vi "Labspec MoveMotor.vi"(6 "Position Name":string, 7 "Modes":T1[](array[typedef]) items=["Value"=0, "Step"=1, "Index"=2, "String"=3, "Calibrate"=4, "Origin"=5, "Stop"=6, "Value to Step"=7, "No Wait"=10, "No Message"=100], 8 "error in":errorcluster, 9 "Position Value":dbl=1.0, 10 "Motor Name":T2=enum."Hole", 11 "Automation Refnum In":refnum<k7>) -> (0 "error out":errorcluster, 2 "MoveID":i32, 3 "Automation Refnum Out":refnum<k7>)   [LabVIEW 2014]
uses:
  MoveMotor Motor Name.ctl
  MoveMotor Mode.ctl
panel:
  in  "Motor type (as in documentation)":u16(ring)=6 items=["Spectro", "Mono", "Grating", "Slit", "Hole", "X", "Y", "Z", "Laser"]
  # "LICENSED MATERIALS – PROPERTY OF IBM\nCopyright IBM Corp. 2016,\nALL RIGHTS RESERVED"
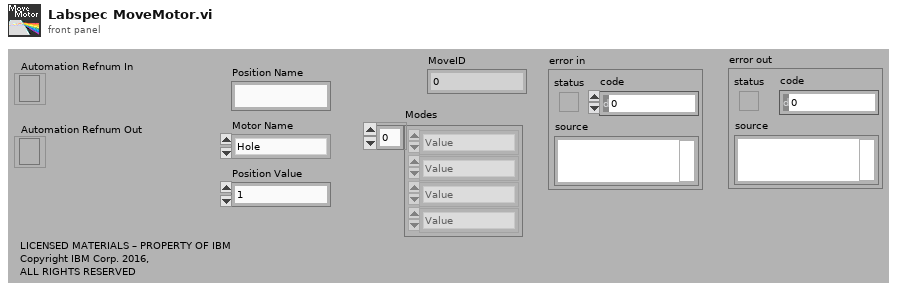
[diagram p1: front panel]
types:
  T1 = typedef "MoveMotor Mode.ctl" = u16
  T2 = typedef "MoveMotor Motor Name.ctl" = enum16{"Spectro", "Premono", "Grating", "Slit", "Hole", "X", "Y", "XT", "YT", "XL", "YL", "Z", "Laser", "Filter", "Objective", "Detector", "Detector Temperature"}
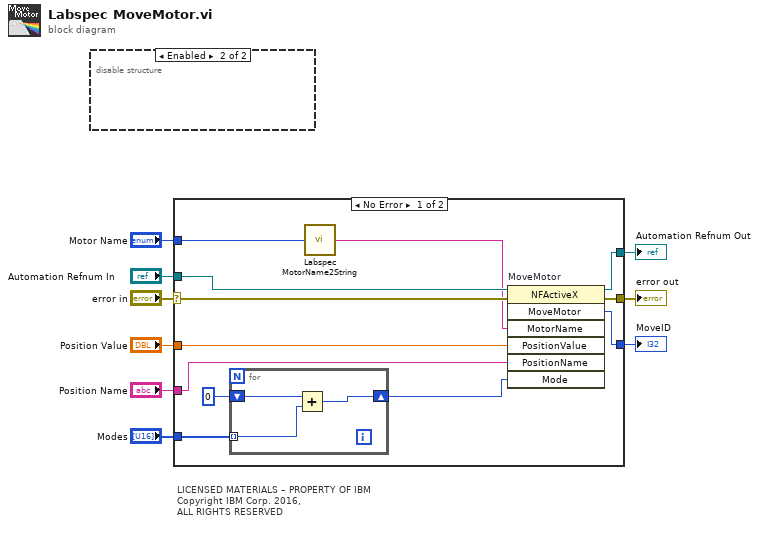
[diagram p0: block diagram]
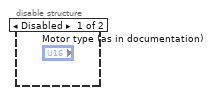
[diagram p2: hidden frame]
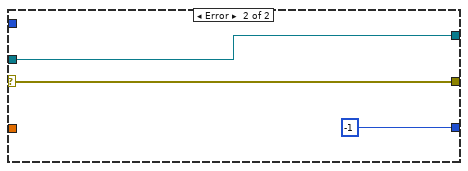
[diagram p3: hidden frame]
diagram:
  # "LICENSED MATERIALS – PROPERTY OF IBM\nCopyright IBM Corp. 2016,\nALL RIGHTS RESERVED"
  n1 = disable-structure shown="Enabled" {
    frame Disabled {
    }
    frame Enabled {
    }
  }
  n2 = case shown="No Error" "error in" {
    selector: "error in" -> [w15 w25]
    tunnel: "Modes" -> [w12 _]
    tunnel: "Position Name" -> [w21 _]
    tunnel: [w20 -1 ("MoveMotor")] -> w8
    tunnel: "Position Value" -> [w19 _]
    tunnel: "Motor Name" -> [w14 _]
    tunnel: "Automation Refnum In" -> [w18 w27]
    tunnel: [w17 w27] -> w2
    tunnel: [w16 w25] -> w4
    frame No Error {
      n3 = for {
        tunnel: w12 -> [w22] mode=indexing
        shift-right: [w24] -> w10
        shift-left: 0 ("Mode") -> [w23]
        n4 = Add(x=w23, y=w22) -> (x+y=w24:i32)
      }
      n5 = call "Labspec MotorName2String.vi"("Motor Name"=w14) -> ("PositionName"=w13:string)
      n6 = invoke on="MoveMotor" class="NFActiveX" method="MoveMotor"(reference=w18, error in=w15, "MotorName"=w13, "PositionValue"=w19, "PositionName"=w21, "Mode"=w10) -> (reference out=w17:refnum<k7>, error out=w16:errorcluster, "MoveMotor"=w20:i32)  [unwired: 1 in, 4 out]
    }
    frame Error {
    }
  }
  "error out" <- w4
  "Automation Refnum Out" <- w2
  "MoveID" <- w8
